vi "GetWaferData.vi"(8 "error in (no error)":errorcluster, 11 "LotData in":refnum<class "LotData.lvclass">) -> (0 "error out":errorcluster, 3 "LotData out":refnum<class "LotData.lvclass">)   [LabVIEW 2012, in "LotData.lvclass"]
uses:
  LotData.lvclass
  Controls/TestData.ctl
  <vilib>/addons/database/Auxilliary.llb/DB Tools Parameter Info.ctl
  <vilib>/addons/database/Auxilliary.llb/DB Tools DataTypes.ctl
  <vilib>/addons/database/Auxilliary.llb/DB Tools Parameter Dir.ctl
  LotData.lvclass/LotData.ctl
  Controls/TestArea.ctl
  <vilib>/addons/database/Connection.llb/DB Tools Open Connec (Path).vi
  <vilib>/addons/database/Command.llb/Cmd Set Parameter Value (C).vi
  <vilib>/addons/database/Command.llb/Cmd Execute.vi
  <vilib>/addons/database/Recordset.llb/Rec Fetch Recordset Data (CR).vi
  <vilib>/addons/database/Recordset.llb/Rec Destroy - Command.vi
  <vilib>/addons/database/Command.llb/Cmd Delete.vi
  <vilib>/addons/database/_DB Variant To Data/Database Variant To Data.xnode
  <vilib>/addons/database/NI_Database_API.lvlib
panel:
  out "Array":T1[](array[typedef]) {"50mA Data"."Current,mA" format="%_6g"; "50mA Data"."WL" format="%_6g"; "50mA Data"."Voltage" format="%_6g"; "50mA Data"."Power" format="%_6g"; "20mA Data"."Reverse" format="%#_3g"; "20mA Data"."Current,mA" format="%_6g"; "20mA Data"."Knee Current" format="%#_3g"; "20mA Data"."WL" format="%_6g"; "20mA Data"."Voltage" format="%_6g"; "20mA Data"."Power" format="%_5g"}
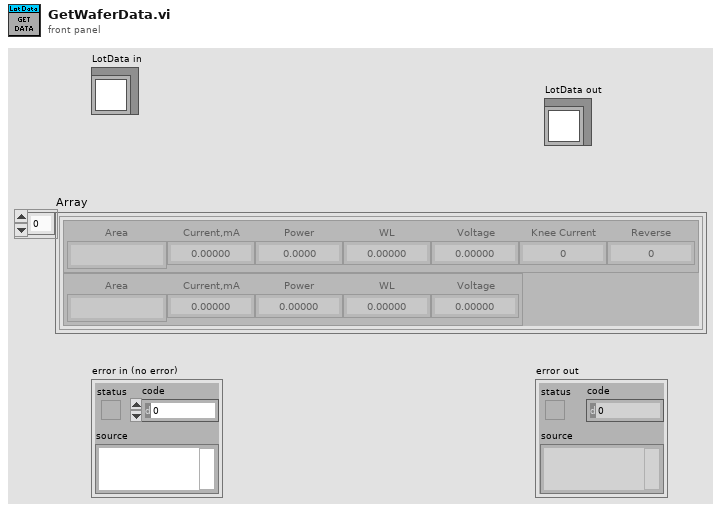
[diagram p1: front panel]
types:
  T1 = typedef "TestData.ctl" = cluster{"20mA Data":cluster{"Area":string, "Current,mA":dbl, "Power":dbl, "WL":dbl, "Voltage":dbl, "Knee Current":dbl, "Reverse":dbl}, "50mA Data":cluster{"Area":string, "Current,mA":dbl, "Power":dbl, "WL":dbl, "Voltage":dbl}}
  T2 = typedef "NI_Database_API.lvlib/DB Tools Parameter Info.ctl" = cluster{"parameter name":string, "type":T3, "direction":T4, "value":variant}
  T3 = typedef "NI_Database_API.lvlib/DB Tools DataTypes.ctl" = enum16{"String", "Long (I32)", "Single (SGL)", "Double (DBL)", "Date/Time", "Binary"}
  T4 = typedef "NI_Database_API.lvlib/DB Tools Parameter Dir.ctl" = enum32{"Input", "Output", "Input/Output", "Return Value"}
  T5 = cluster{"Area":string, "Current,mA":dbl, "Power":dbl, "WL":dbl, "Voltage":dbl, "Knee Current":dbl, "Reverse":dbl}
  T6 = typedef "TestArea.ctl" = string
  T7 = typedef "NI_Database_API.lvlib/Conn ObjectReference.ctl" = refnum<k1>
  T8 = typedef "NI_Database_API.lvlib/Cmd ObjectReference.ctl" = refnum<k1>
  T9 = typedef "NI_Database_API.lvlib/Cmd-Rec Object Reference.ctl" = refnum<k1>
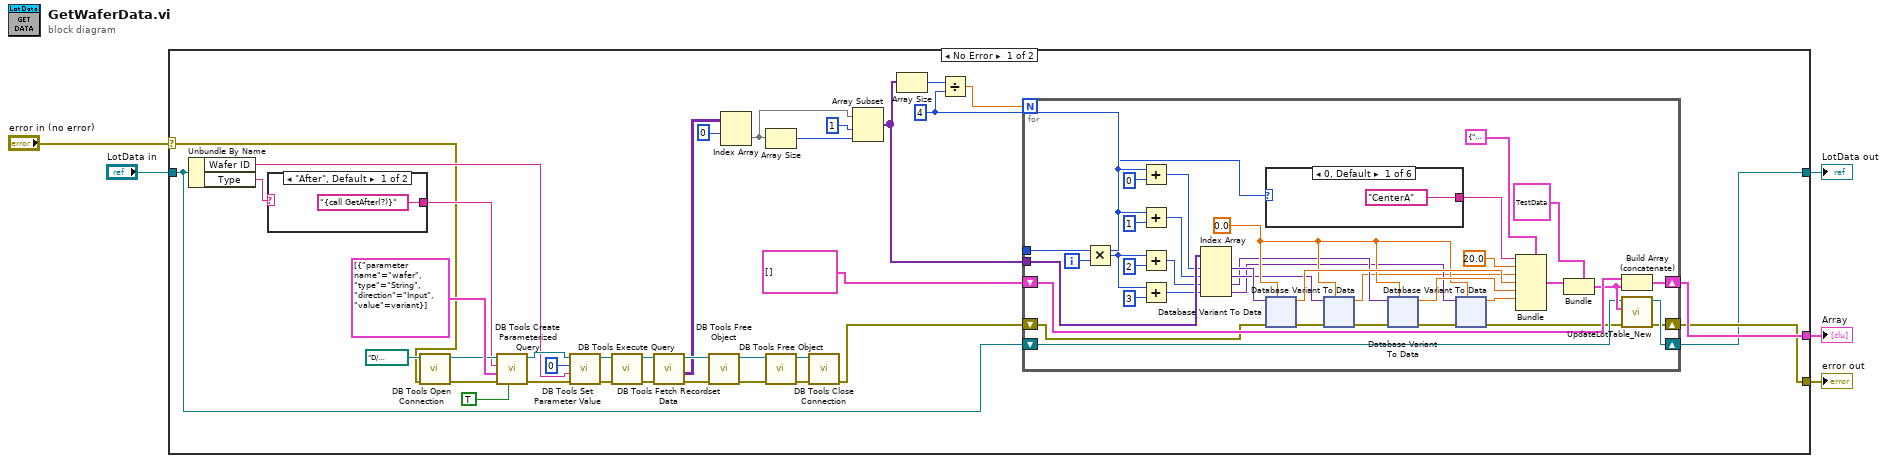
[diagram p0: block diagram]
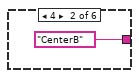
[diagram p2: hidden frame]
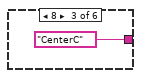
[diagram p3: hidden frame]
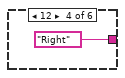
[diagram p4: hidden frame]
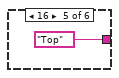
[diagram p5: hidden frame]
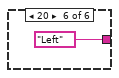
[diagram p6: hidden frame]
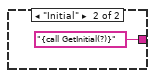
[diagram p7: hidden frame]
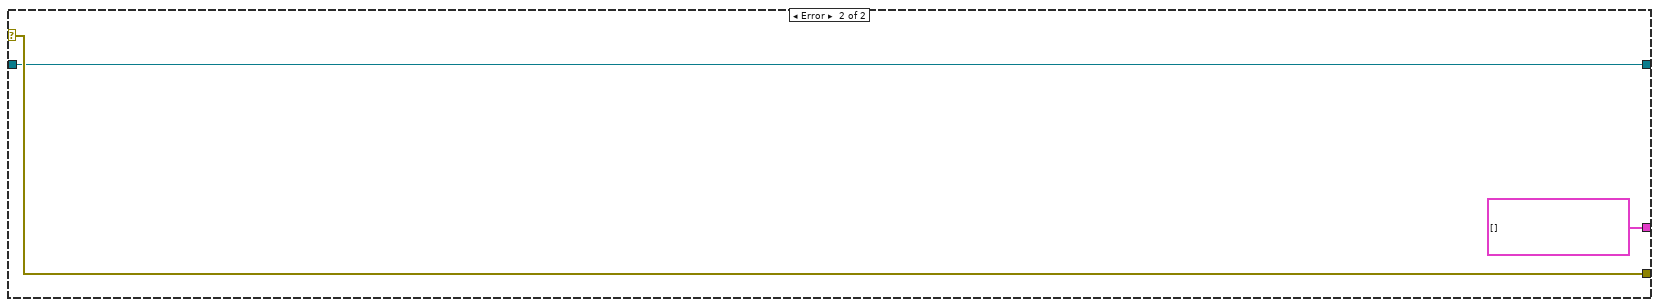
[diagram p8: hidden frame]
diagram:
  n1 = case shown="No Error" "error in (no error)" {
    selector: "error in (no error)" -> [w6 w218]
    tunnel: [w9 w218] -> w2
    tunnel: [w7 w217] -> w1
    tunnel: "LotData in" -> [w8 w217]
    tunnel: [w10 T1[] []] -> w3
    frame No Error {
      w14 = 4 ("y")
      n2 = Unbundle By Name(w8) -> ("Wafer ID"=w12:string, "Type"=w42:string)
      n3 = case shown="\"After\", Default" w42 {
        tunnel: ["{call GetAfter(?)}" ("SQL query") "{call GetInitial(?)}" ("SQL query")] -> w11
        frame "After", Default {
        }
        frame "Initial" {
        }
      }
      n4 = call-poly <vilib>:"DB Tools Open Connection.vi"("error in (no error)"=w6, "connection information"=path "D:/Program Files (x86)/National Instruments/LabVIEW 2012/Database/epiDataLink.udl") -> ("error out"=w37:errorcluster, "connection reference"=w38:T7)  [unwired: 6 in]
      n5 = call <vilib>:"DB Tools Create Parameterized Query.vi"("stored procedure? (F)"=TRUE, "error in (no error)"=w37, "parameters"=T2[] [{"parameter name"="wafer", "type"=enum."String", "direction"=enum."Input", "value"=variant}], "SQL query"=w11, "connection reference"=w38) -> ("error out"=w35:errorcluster, "command reference"=w34:T8)  [unwired: 2 in, 1 out]
      n6 = call-poly <vilib>:"DB Tools Set Parameter Value.vi"("error in (no error)"=w35, "value"=w12, "parameter index"=0, "command reference"=w34) -> ("error out"=w31:errorcluster, "command reference out"=w32:T8)  [unwired: 4 in]
      n7 = call-poly <vilib>:"DB Tools Execute Query.vi"("error in (no error)"=w31, "command reference"=w32) -> ("error out"=w26:errorcluster, "command-recordset reference"=w27:T9)  [unwired: 6 in]
      n8 = call-poly <vilib>:"DB Tools Fetch Recordset Data.vi"("error in (no error)"=w26, "command-recordset reference"=w27) -> ("error out"=w25:errorcluster, "recordset data"=w23:variant[][], "command-recordset reference out"=w24:T9)  [unwired: 3 in]
      n9 = call-poly <vilib>:"DB Tools Free Object.vi"("error in (no error)"=w25, "command-recordset reference"=w24) -> ("error out"=w33:errorcluster, "command reference"=w28:T8)  [unwired: 8 in]
      n10 = Index Array(array=w23, index (row)=0) -> (element=w18:variant[])  [unwired: 1 in]
      n11 = Array Size(array=w18) -> (size(s)=w16:i32)
      n12 = call-poly <vilib>:"DB Tools Free Object.vi"("error in (no error)"=w33, "command reference"=w28) -> ("error out"=w29:errorcluster, "connection reference"=w30:T7)  [unwired: 8 in]
      n13 = call <vilib>:"DB Tools Close Connection.vi"("error in (no error)"=w29, "connection reference"=w30) -> ("error out"=w19:errorcluster)  [unwired: 5 in]
      n14 = Array Subset(array=w18, index=1, length=w16) -> (w17:variant[])
      n15 = Array Size(array=w17) -> (size(s)=w15:i32)
      n16 = Divide(x=w15, y=w14) -> (x/y=w13:dbl)
      n17 = for {
        N: w13 -> [_]
        tunnel: w17 -> [w68]
        shift-right: [w77] -> w10
        shift-left: T1[] [] -> [w79]
        shift-right: [w43] -> w9
        shift-left: w19 -> [w56]
        tunnel: w14 -> [w55]
        shift-right: [w45] -> w7
        shift-left: w8 -> [w46]
        i -> [w78]
        w69 = 0.0
        n18 = Multiply(x=w55, y=w78) -> (x*y=w53:i32)
        n19 = Add(x=w53, y=0 ("index")) -> (x+y=w67:i32)
        n20 = Add(x=w53, y=1 ("index")) -> (x+y=w66:i32)
        n21 = Add(x=w53, y=2 ("index")) -> (x+y=w65:i32)
        n22 = Add(x=w53, y=3 ("index")) -> (x+y=w64:i32)
        n23 = Index Array(array=w68, index #1=w67, index #2=w66, index #3=w65, index #4=w64) -> (element #1=w63:variant, element #2=w61:variant, element #3=w60:variant, element #4=w59:variant)
        n24 = case shown="0, Default" w53 {
          tunnel: [T6 "CenterA" ("Area") T6 "CenterB" ("Area") T6 "CenterC" ("Area") T6 "Right" ("Area") T6 "Top" ("Area") T6 "Left" ("Area")] -> w52
          frame 0, Default {
          }
          frame 4 {
          }
          frame 8 {
          }
          frame 12 {
          }
          frame 16 {
          }
          frame 20 {
          }
        }
        n25 = xnode "Database Variant To Data"("database variant"=w63, "error in (no error)"=w56, "type"=w69) -> ("data"=w72:dbl, "error out"=w62:errorcluster)
        n26 = xnode "Database Variant To Data"("database variant"=w61, "error in (no error)"=w62, "type"=w69) -> ("data"=w54:dbl, "error out"=w58:errorcluster)
        n27 = xnode "Database Variant To Data"("database variant"=w60, "error in (no error)"=w58, "type"=w69) -> ("data"=w71:dbl, "error out"=w57:errorcluster)
        n28 = xnode "Database Variant To Data"("database variant"=w59, "error in (no error)"=w57, "type"=w69) -> ("data"=w70:dbl, "error out"=w44:errorcluster)
        n29 = Bundle(cluster=T5 {"Area"="", "Current,mA"=0.0, "Power"=0.0, "WL"=0.0, "Voltage"=0.0, "Knee Current"=0.0, "Reverse"=0.0} ("20mA Data"), "Area"=w52, "Current,mA"=20.0, "Power"=w54, "WL"=w72, "Voltage"=w71, "Knee Current"=w70) -> (w48:T5)  [unwired: 1 in]
        n30 = Bundle(cluster=T1 {"20mA Data"={"Area"="Left", "Current,mA"=0.0, "Power"=333.0, "WL"=277.2, "Voltage"=11.8, "Knee Current"=6.4, "Reverse"=0.0}, "50mA Data"={"Area"="", "Current,mA"=0.0, "Power"=0.0, "WL"=0.0, "Voltage"=0.0}} ("input cluster"), "20mA Data"=w48) -> (w47:T1)  [unwired: 1 in]
        n31 = Build Array (concatenate)(w79, w47) -> (w77:T1[])
        n32 = call-dynamic "UpdateLotTable_New.vi"("error in (no error)"=w44, "input cluster"=w47, "LotData in"=w46) -> ("error out"=w43:errorcluster, "LotData out"=w45:refnum<class "LotData.lvclass">)  [unwired: 7 in]
      }
    }
    frame Error {
    }
  }
  "error out" <- w2
  "LotData out" <- w1
  "Array" <- w3
